vi "Get Positionner error _ controller state_TS.vi"(8 "error in (no error)":errorcluster caption="entrée d'erreur (pas d'erreur)", 10 "controllerAddress":i32, 11 "SMC100 in":refnum<k24>) -> (0 "error out":errorcluster caption="sortie d'erreur", 1 "errstring":string, 2 "controllerState":string, 3 "SMC100 out":refnum<k24>, 4 "errorCode":string)   [LabVIEW 2024, in "SMC100.lvlib"]
uses:
  SMC100.lvlib
  Newport.SMC100.CommandInterface
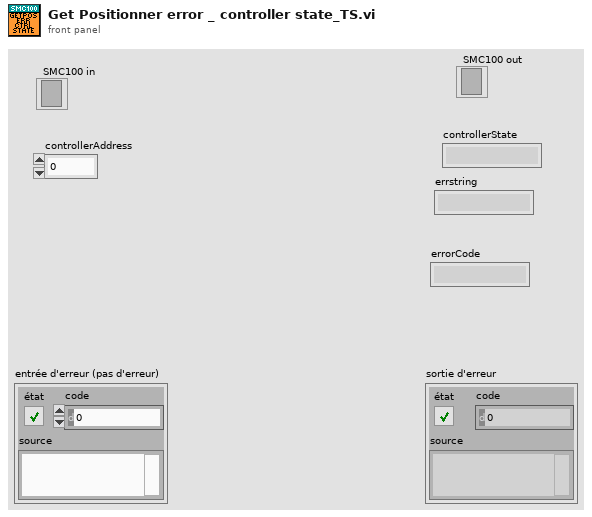
[diagram p1: front panel]
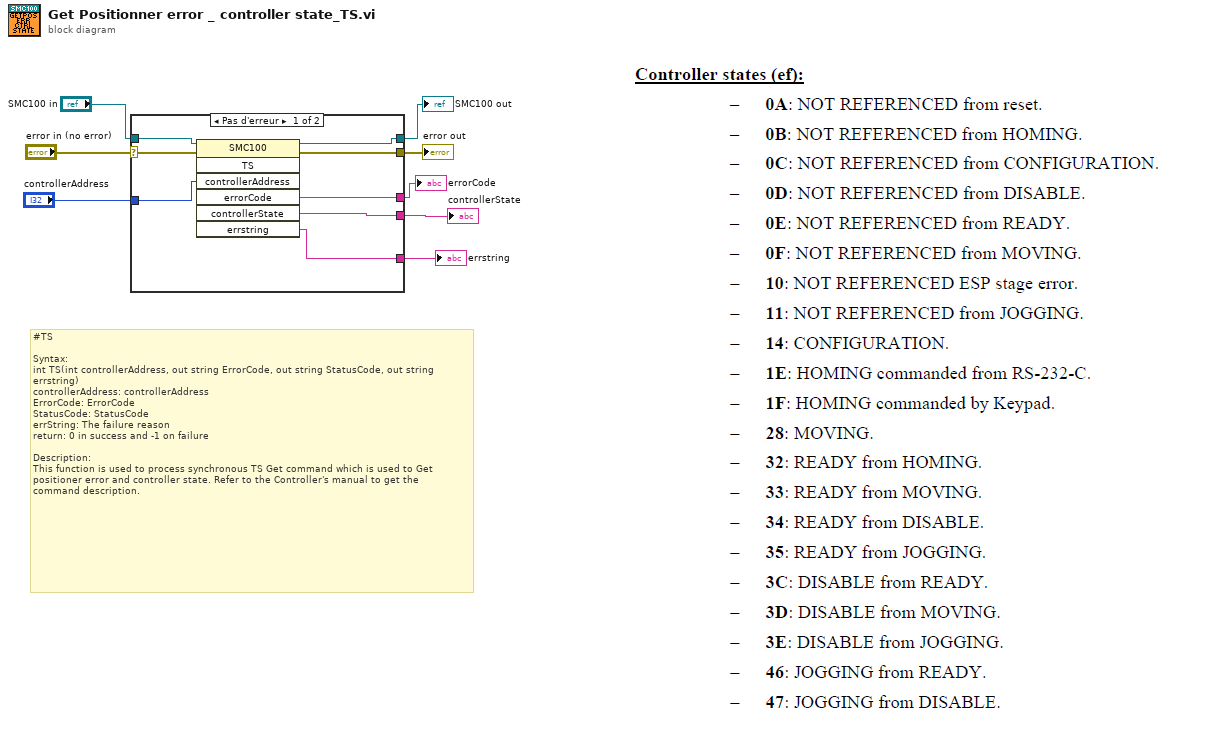
[diagram p0: block diagram]
diagram:
  # "#TS\n\nSyntax:\nint TS(int controllerAddress, out string ErrorCode, out string StatusCode, out string\nerrstring)\ncontrollerAddress: controllerAddress\nErrorCode: ErrorCode\nStatusCode: StatusCode\nerrString: The failure reason\nreturn: 0 in success and -1 on failure\n\nDescription:\nThis function is used to process synchronous TS Get command which is used to Get\npositioner error and controller state. Refer to the Controller's manual to get the\ncommand description."
  n1 = case shown="Pas d'erreur" "error in (no error)" {
    selector: "error in (no error)" -> [w16 w17]
    tunnel: [w15 w17] -> w7
    tunnel: "SMC100 in" -> [w14 w18]
    tunnel: [w13 w18] -> w5
    tunnel: "controllerAddress" -> [w12 _]
    tunnel: [w11 _] -> w3
    tunnel: [w10 _] -> w2
    tunnel: [w9 _] -> w1
    frame No Error {
      n2 = invoke class="SMC100" method="TS"(reference=w14, error in=w16, "controllerAddress"=w12) -> (reference out=w13:refnum<k24>, error out=w15:errorcluster, "errorCode"=w10:string, "controllerState"=w11:string, "errstring"=w9:string)  [unwired: 4 in, 2 out]
    }
    frame Error {
    }
  }
  "error out" <- w7
  "SMC100 out" <- w5
  "controllerState" <- w3
  "errorCode" <- w2
  "errstring" <- w1
